vi "Create System Log.vi"(8 "error in":errorcluster, 10 "TimeStamp":string, 11 "File IO Data":T1={"System Log File"=path "", "Data File"=path "", "Work Order Folder"=path "", "Report Template Folder"=path "", "Report Folder"=path "", "Report File"=path "", "APU Setup Folder"=path "", "Testing State"=FALSE, "Recording State"=FALSE, "Test Information"={"APU Part Number:"="", "Model:"="", "Serial Number:"="", "Customer:"="", "Work Order:"="", "Pre or Post SB"="", "Run Count"=0, "APU Selected"="<Select>"}, "Crash Log Data"=[], "Group Name"="", "APU Setup"={"Sensor Info"=[], "Variables"=[], "CMM Table 106"=[], "CMM Table 106B "=[], "Accel Config"=[], "Report Sheet 1"=[], "Report Sheet 2"=[], "Report Sheet 3"=[]}, "ChannelTagsToLog"=[], "report ref"=refnum, "APU Setup File"=path "", "RunTimes"=[], "ReportHeader"=[]} {"Test Information"."Run Count" min=0 step=1}) -> (0 "error out":errorcluster, 3 "File IO Data":T1={"System Log File"=path "", "Data File"=path "", "Work Order Folder"=path "", "Report Template Folder"=path "", "Report Folder"=path "", "Report File"=path "", "APU Setup Folder"=path "", "Testing State"=FALSE, "Recording State"=FALSE, "Test Information"={"APU Part Number:"="", "Model:"="", "Serial Number:"="", "Customer:"="", "Work Order:"="", "Pre or Post SB"="", "Run Count"=0, "APU Selected"="<Select>"}, "Crash Log Data"=[], "Group Name"="", "APU Setup"={"Sensor Info"=[], "Variables"=[], "CMM Table 106"=[], "CMM Table 106B "=[], "Accel Config"=[], "Report Sheet 1"=[], "Report Sheet 2"=[], "Report Sheet 3"=[]}, "ChannelTagsToLog"=[], "report ref"=refnum, "APU Setup File"=path "", "RunTimes"=[], "ReportHeader"=[]} {"Test Information"."Run Count" min=0 step=1})   [LabVIEW 2018, in "File IO.lvlib"]
doc: "Use the Test Information to create a new TDMS file."
uses:
  File IO.lvlib
  Private Controls/File IO Data.ctl
  <vilib>/Utility/NIReport.llb/NI_report.lvclass
  Controller (Host)/Public Controls/Test Information.ctl
  Controller (Host)/Public VIs/PreorPostSB.ctl
  Controller (Host)/Public Controls/APU Select.ctl
  Top Level/Shared Controls/Analyzed Data Sets.ctl
  Top Level/Shared Controls/All Data Cluster.ctl
  Top Level/Shared Controls/Acq Data.ctl
  Top Level/Shared Controls/APU Setup File.ctl
  <vilib>/Utility/file.llb/Write Delimited Spreadsheet (string).vi
  Testing UI 1/Testing UI 1.lvlib
  Controller (Host)/Controller (Host).lvlib
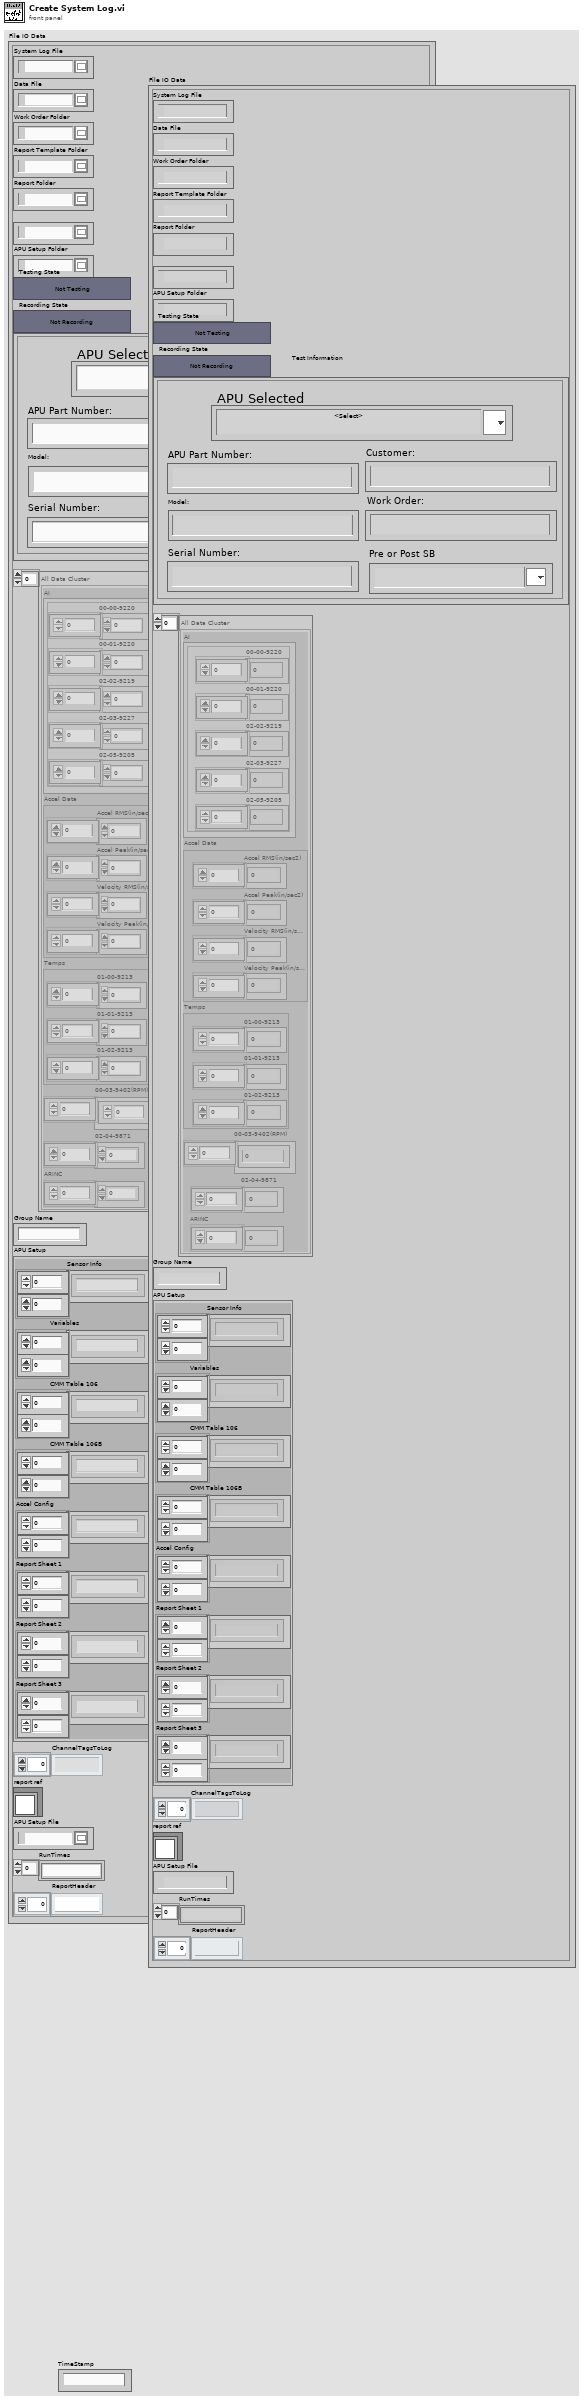
[diagram p1: front panel]
types:
  T1 = typedef "File IO.lvlib/File IO Data.ctl" = cluster{"System Log File":path, "Data File":path, "Work Order Folder":path, "Report Template Folder":path, "Report Folder":path, "Report File":path, "APU Setup Folder":path, "Testing State":bool, "Recording State":bool, "Test Information":T2, "Crash Log Data":T5, "Group Name":string, "APU Setup":T8, "ChannelTagsToLog":string[], "report ref":refnum<class "NI_report.lvclass">, "APU Setup File":path, "RunTimes":string[], "ReportHeader":string[]}
  T2 = typedef "Controller (Host).lvlib/Test Information.ctl" = cluster{"APU Part Number:":string, "Model:":string, "Serial Number:":string, "Customer:":string, "Work Order:":string, "Pre or Post SB":T3, "Run Count":i32, "APU Selected":T4}
  T3 = typedef "Controller (Host).lvlib/PreorPostSB.ctl" = string
  T4 = typedef "Controller (Host).lvlib/APU Select.ctl" = string
  T5 = typedef "Analyzed Data Sets.ctl" = T6[]
  T6 = typedef "All Data Cluster.ctl" = cluster{"AI":T7, "Accel Data":cluster{"Accel RMS(in/sec2)":dbl[], "Accel Peak(in/sec2)":dbl[], "Velocity RMS(in/sec)":dbl[], "Velocity Peak(in/sec)":dbl[]}, "Temps":cluster{"01-00-9213":dbl[], "01-01-9213":dbl[], "01-02-9213":dbl[]}, "00-03-9402(RPM)":dbl[], "02-04-9871":dbl[], "ARINC":sgl[]}
  T7 = typedef "Acq Data.ctl" = cluster{"00-00-9220":dbl[], "00-01-9220":dbl[], "02-02-9219":dbl[], "02-03-9227":dbl[], "02-05-9205":dbl[]}
  T8 = typedef "APU Setup File.ctl" = cluster{"Sensor Info":string[][], "Variables":string[][], "CMM Table 106":string[][], "CMM Table 106B ":string[][], "Accel Config":string[][], "Report Sheet 1":string[][], "Report Sheet 2":string[][], "Report Sheet 3":string[][]}
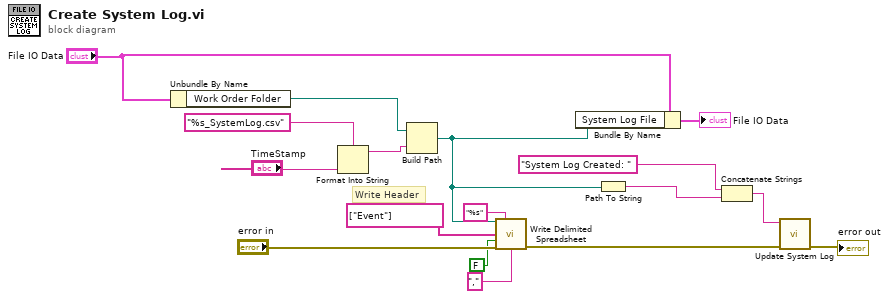
[diagram p0: block diagram]
diagram:
  # "Write Header"
  n1 = Unbundle By Name("File IO Data") -> ("Work Order Folder"=w15:path)
  n2 = Format Into String(format string="%s_SystemLog.csv", "TimeStamp") -> (resulting string=w13:string)  [unwired: 2 in, 1 out]
  n3 = Build Path(base path=w15, name or relative path=w13) -> (appended path=w2:path)
  n4 = call-poly <vilib>:"Write Delimited Spreadsheet.vi"("file path (dialog if empty)"=w2, "format (%s)"="%s" ("format (%.3f)"), "1D data"=string[] ["Event"] ("format (%.3f)"), "append to file? (new file:F)"=FALSE, "error in (no error)"="error in", "delimiter (\\t)"="," ("delimiter (\\t)")) -> ("error out"=w3:errorcluster)  [unwired: 8 in, 1 out]
  n5 = Bundle By Name(cluster="File IO Data", "System Log File"=w2) -> (→"File IO Data":T1)
  n6 = Path To String(path=w2) -> (string=w5:string)
  n7 = Concatenate Strings("System Log Created: " ("Message"), w5) -> (w4:string)
  n8 = call "Update System Log.vi"("error in"=w3, "Message"=w4) -> ("error out"=→"error out":errorcluster)  [unwired: 9 in]
